vi "RTcodeRemoveLater.vi"() -> ()   [LabVIEW 2018]
uses:
  <vilib>/FPGAPlugInAG/cRIO-9049/niLvFpga_Open_cRIO-9049.vi
  <vilib>/rvi/interface/common/dynamic/niFpgaDynamicAddResources.vi
  <vilib>/Utility/error.llb/Error Cluster From Error Code.vi
  <vilib>/rvi/errors/niLvFpgaAdjustHostInterfaceError.vi
  <vilib>/FPGAPlugInAG/Dynamic/niLvFpga_Close_Dynamic.vi
  <vilib>/rvi/interface/nirviOpenFPGA/nirviOpenFPGA.xnode
  fpgaInterface/NiFpga_mainFPGA.lvbitx
  <vilib>/rvi/interface/nirviReadWriteControl/nirviReadWriteControl.xnode
  <vilib>/rvi/interface/nirviMethod/nirviMethod.xnode
  <vilib>/rvi/interface/nirviCloseFPGA/nirviCloseFPGA.xnode
  <vilib>/FPGAPlugInAG/Dynamic/niLvFpga_ReadFifo_Dynamic.vi
  <vilib>/rvi/errors/niLvFpgaMergeErrorWithErrorCode.vi
  <vilib>/rvi/interface/Simulation/niFpgaSimulationCallBeginRW.vi
  NiFpgaLv.dll
panel:
  in  "error in":errorcluster
  out "error out":errorcluster
  in  "waitInMs":u32=1000
  out "Data":u16[](array[numeric])
  in  "milliseconds to wait":u32=500
  out "dataFifoFull":bool
  in  "stop":bool
  out "Numeric 9":u16
  out "Numeric 8":u16
  out "Numeric 7":u16
  out "Numeric 6":u16
  out "Numeric 5":u16
  out "Numeric 4":u16
  out "Numeric 3":u16
  out "Numeric 2":u16
  out "Numeric":u16
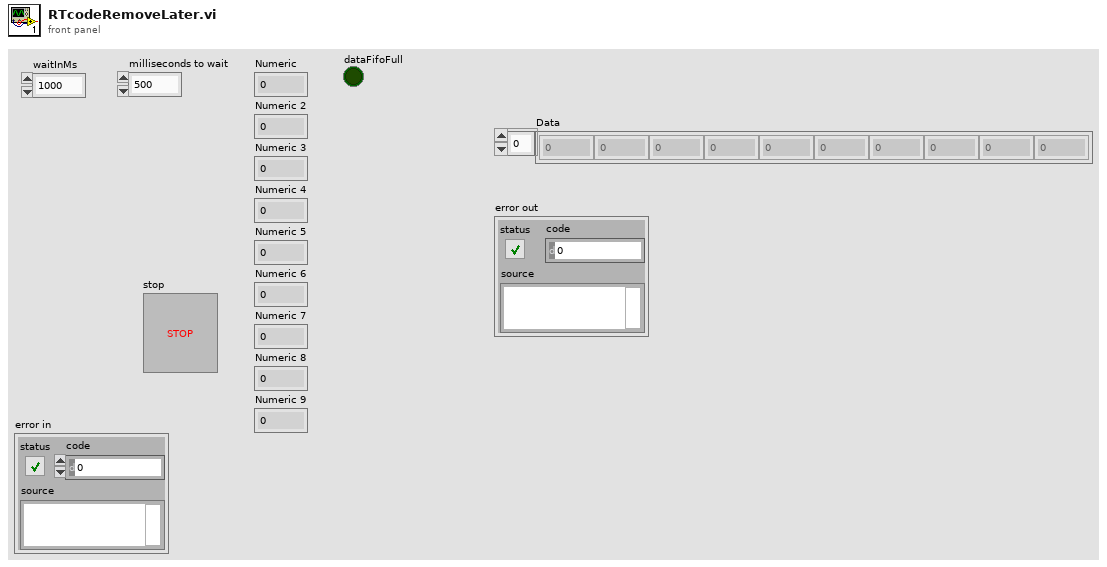
[diagram p1: front panel]
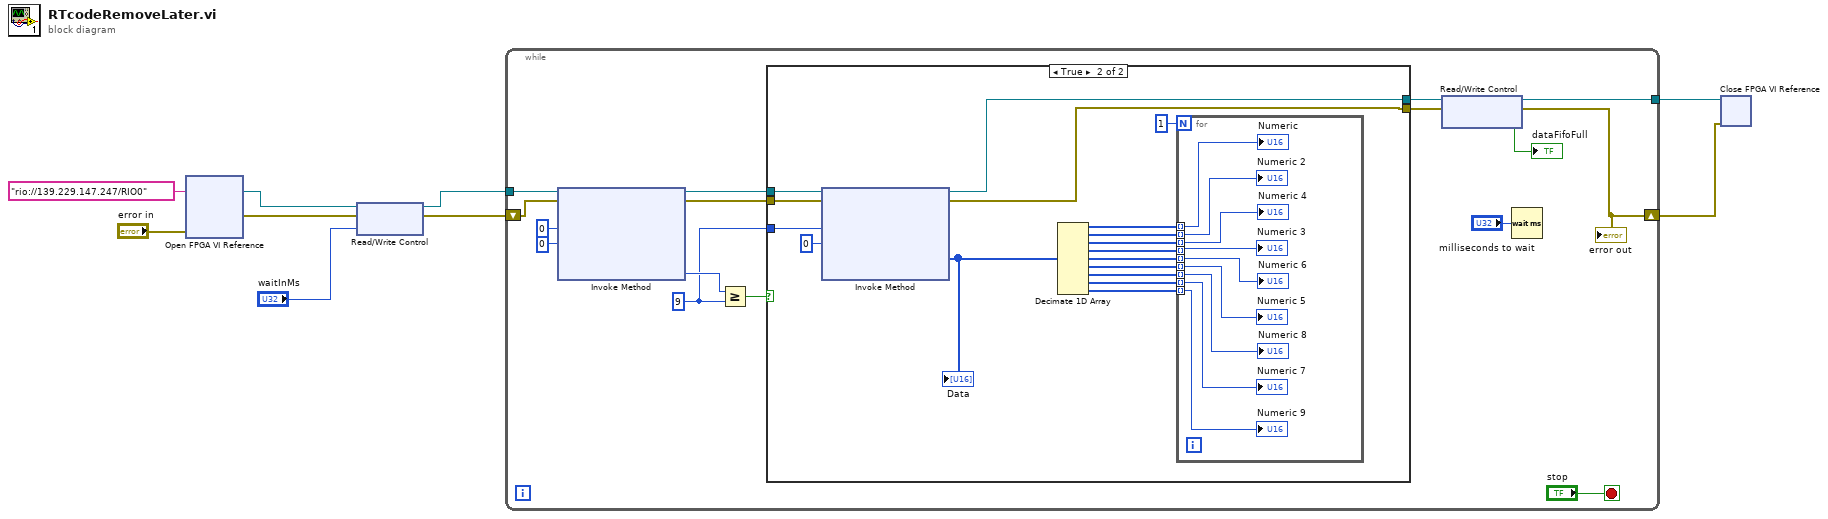
[diagram p0: block diagram]
diagram:
  n1 = xnode "Open FPGA VI Reference"("error in"="error in", "resource name"=tag "rio://139.229.147.247/RIO0") -> ("FPGA VI Reference Out"=w3:refnum<k20>, "error out"=w2:errorcluster)
  n2 = xnode "Read/Write Control"("FPGA VI Reference In"=w3, "error in"=w2, "waitInMs"="waitInMs") -> ("FPGA VI Reference Out"=w6:refnum<k20>, "error out"=w7:errorcluster)
  n3 = while {
    tunnel: w6 -> [w25]
    tunnel: [w13] -> w9
    shift-right: [w12] -> w8
    shift-left: w7 -> [w18]
    stop <- "stop" stop-if-true
    w17 = u32 9 ("y")
    n4 = xnode "Invoke Method"("FPGA VI Reference In"=w25, "error in"=w18, "Number of Elements"=u32 0, "Timeout (ms)"=0) -> ("FPGA VI Reference Out"=w20:refnum<k20>, "error out"=w19:errorcluster, "Elements Remaining"=w22:u32)  [unwired: 1 out]
    n5 = Greater Or Equal?(x=w22, y=w17) -> (x >= y?=w21:bool)
    n6 = case shown="True" w21 {
      tunnel: w20 -> [w27 w44]
      tunnel: w19 -> [w26 w43]
      tunnel: w17 -> [_ w41]
      tunnel: [w27 w30] -> w15
      tunnel: [w26 w29] -> w14
      frame False {
      }
      frame True {
        n7 = xnode "Invoke Method"("FPGA VI Reference In"=w44, "error in"=w43, "Number of Elements"=w41, "Timeout (ms)"=0) -> ("FPGA VI Reference Out"=w30:refnum<k20>, "error out"=w29:errorcluster, "Data"=w28:u16[])  [unwired: 1 out]
        "Data" <- w28
        n8 = Decimate 1D Array(w28) -> (w39:u16[], w38:u16[], w37:u16[], w36:u16[], w35:u16[], w34:u16[], w33:u16[], w32:u16[], w31:u16[])
        n9 = for {
          N: 1 -> [_]
          tunnel: w39 -> [w53] mode=indexing
          tunnel: w38 -> [w52] mode=indexing
          tunnel: w37 -> [w51] mode=indexing
          tunnel: w36 -> [w50] mode=indexing
          tunnel: w35 -> [w49] mode=indexing
          tunnel: w34 -> [w48] mode=indexing
          tunnel: w33 -> [w47] mode=indexing
          tunnel: w32 -> [w46] mode=indexing
          tunnel: w31 -> [w45] mode=indexing
          "Numeric" <- w53
          "Numeric 2" <- w52
          "Numeric 4" <- w51
          "Numeric 3" <- w50
          "Numeric 6" <- w49
          "Numeric 5" <- w48
          "Numeric 8" <- w47
          "Numeric 7" <- w46
          "Numeric 9" <- w45
        }
      }
    }
    n10 = xnode "Read/Write Control"("FPGA VI Reference In"=w15, "error in"=w14) -> ("FPGA VI Reference Out"=w13:refnum<k20>, "error out"=w12:errorcluster, "dataFifoFull"=→"dataFifoFull":bool)
    "error out" <- w12
    n11 = Wait (ms)(milliseconds to wait="milliseconds to wait") -> ()  [unwired: 1 out]
  }
  n12 = xnode "Close FPGA VI Reference"("FPGA VI Reference In"=w9, "error in"=w8) -> ()  [unwired: 1 out]
